vi "FPGA PWM Out 1ch.vi"(0 "PWM Params":T1={"Pulse Length (Ticks)"=20000, "Pulse Period (Ticks)"=40000, "Ao (Int)"=16384, "Seq 1 (High)"=FALSE, "Seq 2 (Low)"=FALSE}) -> ()   [LabVIEW 2012]
uses:
  <vilib>/rvi/eio/common/nirviEmuTemplateMethod_errors.vi
  <vilib>/eio/EIONode/EIONode.xnode
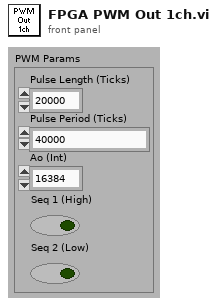
[diagram p1: front panel]
types:
  T1 = cluster{"Pulse Length (Ticks)":u32, "Pulse Period (Ticks)":u32, "Ao (Int)":i32, "Seq 1 (High)":bool, "Seq 2 (Low)":bool}
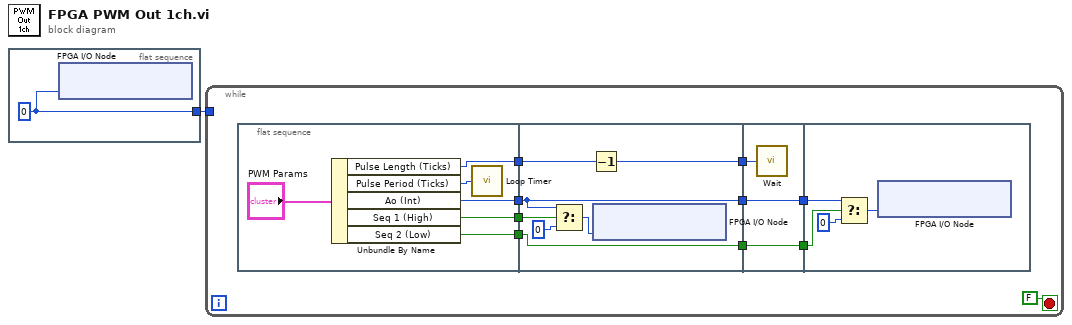
[diagram p0: block diagram]
diagram:
  n1 = flat-sequence {
    tunnel: [w2] -> w1
    frame #0 {
      w2 = i16 0 ("Connector0/AO7")
      n2 = xnode "FPGA I/O Node"("Connector0/AO7"=w2) -> ()  [unwired: 1 in, 1 out]
    }
  }
  n3 = while {
    tunnel: w1 -> [_]
    stop <- FALSE stop-if-true
    n4 = flat-sequence {
      tunnel: [w17] -> w10
      tunnel: [w16] -> w9
      tunnel: [w15] -> w6
      tunnel: [w14] -> w3
      tunnel: [w25] -> w11
      tunnel: w10 -> [w24]
      tunnel: w9 -> [w22]
      tunnel: [w22] -> w7
      tunnel: w6 -> [w21]
      tunnel: [w20] -> w4
      tunnel: w3 -> [w20]
      tunnel: w11 -> [w26]
      tunnel: [w28] -> w8
      tunnel: w7 -> [w28]
      tunnel: [w27] -> w5
      tunnel: w4 -> [w27]
      tunnel: w8 -> [w31]
      tunnel: w5 -> [w30]
      frame #0 {
        n5 = Unbundle By Name("PWM Params") -> ("Pulse Length (Ticks)"=w17:u32, "Pulse Period (Ticks)"=w13:u32, "Ao (Int)"=w16:i32, "Seq 1 (High)"=w15:bool, "Seq 2 (Low)"=w14:bool)
        n6 = call "Loop Timer"("Count(Ticks)"=w13) -> ()  [unwired: 1 out]
      }
      frame #1 {
        n7 = Select(t=w22, s=w21, f=0) -> (s? t:f=w19:i32)
        n8 = Decrement(x=w24) -> (x-1=w25:u32)
        n9 = xnode "FPGA I/O Node"("Connector0/AO7"=w19) -> ()  [unwired: 1 in, 1 out]
      }
      frame #2 {
        n10 = call "Wait"("Count(Ticks)"=w26) -> ()  [unwired: 1 out]
      }
      frame #3 {
        n11 = Select(t=w31, s=w30, f=0) -> (s? t:f=w29:i32)
        n12 = xnode "FPGA I/O Node"("Connector0/AO7"=w29) -> ()  [unwired: 1 in, 1 out]
      }
    }
  }
